vi "GetClusterElementByName(String).vi"(10 "ElementName":string[](array[string]), 11 "Cluster":variant) -> (2 "Found":bool, 3 "ValueOut":string)   [LabVIEW 2013, in "GetClusterElementByName.lvlib"]
uses:
  GetClusterElementByName.lvlib
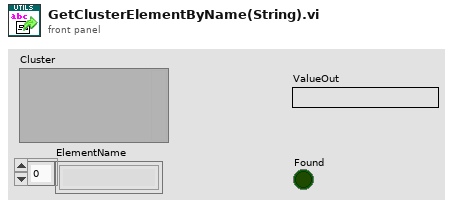
[diagram p1: front panel]
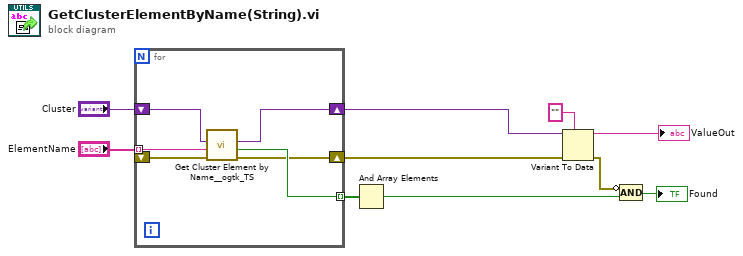
[diagram p0: block diagram]
diagram:
  n1 = for {
    tunnel: "ElementName" -> [w16] mode=indexing
    shift-right: [w15] -> w7
    shift-left: "Cluster" -> [w14]
    tunnel: [w13] -> w8 mode=indexing
    shift-right: [w12] -> w5
    shift-left: _ -> [w11]
    n2 = call "Get Cluster Element by Name__ogtk_TS.vi"("error in (no error)"=w11, "Element Name"=w16, "Cluster"=w14) -> ("error out"=w12:errorcluster, "found?"=w13:bool, "VElement"=w15:variant)  [unwired: 6 in]
  }
  n3 = And Array Elements(Boolean array=w8) -> (logical AND=w4:bool)
  n4 = Variant To Data(error in=w5, type="", Variant=w7) -> (data=→"ValueOut":string, error out=w2:errorcluster)
  n5 = Compound Arithmetic op=AND(invert w2, w4) -> (→"Found":bool)
